vi "GetStateData.vi"(8 "error in (no error)":errorcluster, 11 "PrintF in":refnum<class "PrintF.lvclass">) -> (0 "error out":errorcluster, 1 "Data":string, 2 "State":string, 3 "PrintF out":refnum<class "PrintF.lvclass">)   [LabVIEW 2020, in "UpstreamMsg.lvlib" / "PrintF.lvclass"]
uses:
  PrintF.lvclass
  850c20f9-9062-4f91-a983-530bc3a08ccb.vi
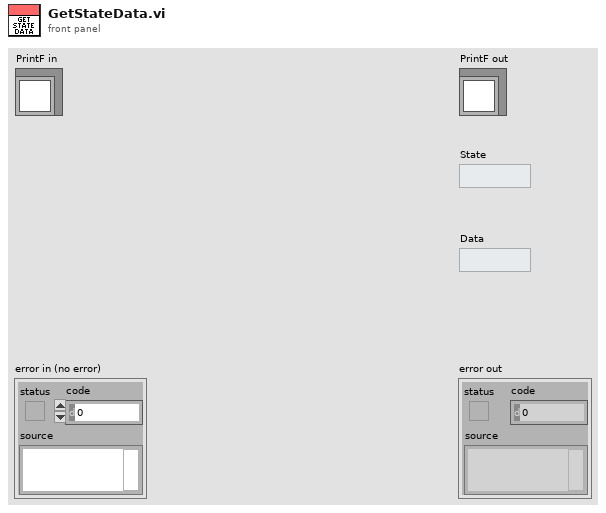
[diagram p1: front panel]
types:
  T1 = typedef "UpstreamMsg.lvlib/PrintF.lvclass/Msg.ctl" = cluster{"TxtColor":cluster{"r":u8, "b":u8, "g":u8}, "LineToPrint":string}
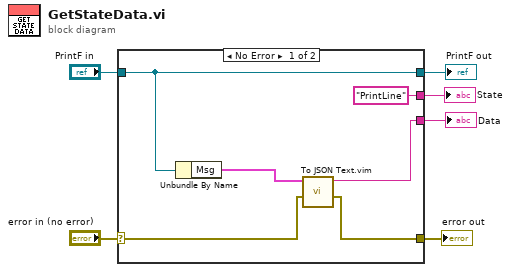
[diagram p0: block diagram]
diagram:
  n1 = case shown="No Error" "error in (no error)" {
    selector: "error in (no error)" -> [w11 w14]
    tunnel: [w9 w14] -> w6
    tunnel: [w8 w13] -> w5
    tunnel: "PrintF in" -> [w8 w13]
    tunnel: [w10 _] -> w2
    tunnel: ["PrintLine" ("State 2") _] -> w1
    frame No Error {
      n2 = Unbundle By Name(w8) -> ("Msg"=w7:T1)
      n3 = call "To JSON Text.vim"("error in (no error)"=w11, "Anything"=w7) -> ("error out"=w9:errorcluster, "<JSON>"=w10:string)  [unwired: 8 in]
    }
    frame Error {
    }
  }
  "error out" <- w6
  "PrintF out" <- w5
  "State" <- w1
  "Data" <- w2
